vi "basic-main.vi"() -> ()   [LabVIEW 2015]
uses:
  states-enum.ctl
  Rack/Methods/Rack-Stop.vi
  Device/Methods/Lickometer-Stop.vi
  Rack/Typedefs/OutputRequest.ctl
  Rack/Typedefs/OutputRequest refnum.ctl
  Rack/Methods/Port drivers/DigitalInput-DataCluster.ctl
  Rack/Typedefs/InputData cluster.ctl
  Device/Typedefs/Lickometer.ctl
  Device/Typedefs/Speaker.ctl
  Device/Typedefs/Juicer.ctl
  Device/Typedefs/Valve.ctl
panel:
  in  "stop":bool
  out "Acc":dbl
  out "Time":dbl format="%#.0f"
  out "Trials":string
  out "Reward Dispensed (uL)":string
  out "Licks":string
  out "CR":string
  out "Miss":string
  out "FA":string
  out "Hits":string
  out "Current State":string
  out "Time Elapsed":dbl format="%<%H:%M:%S>t"
  in  "Tab Control":enum32{"Required", "Optional", "Devices"}(tab)
  in  "Tone Pairs":u16(ring) items=["1: CS+ 10000 Hz, CS- 5000 Hz", "2: CS+ 5800 Hz, CS- 5000 Hz", "3: CS+ 5000 Hz, CS- 10000 Hz", "4: CS+ 8000 Hz, CS- 15000 Hz"]
  in  "Max Time (s)":dbl=3600.0
  in  "Number of trials":string(combo)="200"
  in  "Max number of \nconsecutive trials":string(combo)="3"
  in  "Animal Name":string="Mouse"
  in  "Reward Vol. (uL)":dbl=5.0
  in  "Sequence Directory":path=path "C:/Users/SiapasLab/Desktop/git/wheatley"
  in  "Assay Description":string="Two Choice Audio Discrimination"
  in  "Recording Location":string="BI Room 146"
  in  "Trial delay (ms)":dbl=2000.0
  in  "Punish Time (s)":dbl=25.0
  in  "Trial window (ms)":dbl=3000.0
  in  "ITI lower (s)":dbl=8.0
  in  "ITI upper (s)":dbl=25.0
  in  "Min Licks":i32=1 min=1
  in  "Data Saving Directory":path=path "\\\\CA1-17\\ld8007/anesthesia/data"
  in  "Lickometer":T1={"Settings"={"Min lick duration"=1, "Port name"="bnc_panel.p0.3", "Port index"=0}, "Lick"=FALSE, "Debouncing"={"Semaphore"=refnum, "Lick start"=0}, "OutputRequest event ref"=refnum, "InputData reference"=refnum, "Active hi?"=FALSE}
  out "InputData":T4
  in  "Speaker":T6={"Settings"={"Portname"="BNC_Panel.ao0", "Index"=0, "Timestamp portname"="BNC_Panel.P0.0"}, "OutputRequest event ref"=refnum, "InputData reference"=refnum}
  in  "Juicer":T7={"Mode"=enum."Juice/reward", "Settings"={"Bleed #1 port index"=1, "Bleed #1 port name"="juicer.bleed1", "Bleed #2 port name"="juicer.bleed2", "Bleed #2 port index"=2, "Flush port name"="juicer.flush", "Flush port index"=3, "Purge port name"="juicer.purge", "Purge port index"=0, "Timestamp port name"="dsub_panel.p9.7"}, "OutputRequest event ref"=refnum, "InputData reference"=refnum}
  in  "Valve":T8={"Settings"={"Timestamp port name"="BNC_panel.P0.0", "Port name"="BNC_panel.P0.1", "Port index"=4}, "OutputRequest event ref"=refnum, "InputData reference"=refnum, "Default length (ms)"=100}
  # "(must be on same NI card)"
  # "(must be on same NI card)"
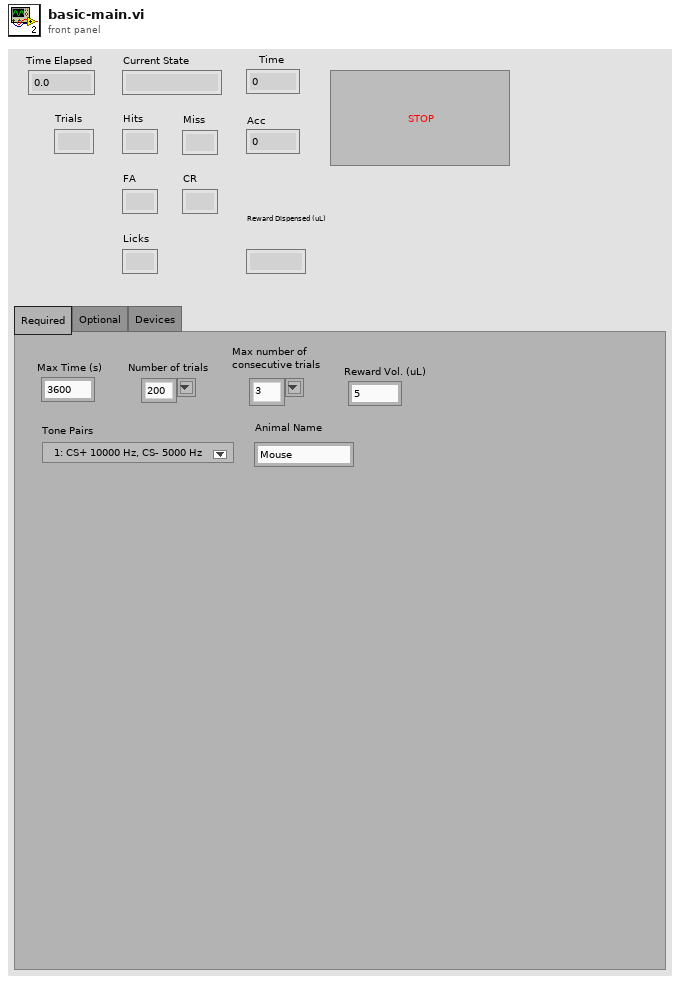
[diagram p1: front panel]
types:
  T1 = typedef "Lickometer.ctl" = cluster{"Settings":cluster{"Min lick duration":u32, "Port name":string, "Port index":i32}, "Lick":bool, "Debouncing":cluster{"Semaphore":T2, "Lick start":u32}, "OutputRequest event ref":T3, "InputData reference":refnum<vi>, "Active hi?":bool}
  T2 = typedef "Semaphore RefNum" = refnum<k1>
  T3 = typedef "OutputRequest refnum.ctl" = refnum<user-event>
  T4 = typedef "InputData cluster.ctl" = cluster{"DigitalInput":T5}
  T5 = typedef "DigitalInput-DataCluster.ctl" = cluster{"Falling":bool[], "Rising":bool[], "State":bool[]}
  T6 = typedef "Speaker.ctl" = cluster{"Settings":cluster{"Portname":string, "Index":i32, "Timestamp portname":string}, "OutputRequest event ref":T3, "InputData reference":refnum<vi>}
  T7 = typedef "Juicer.ctl" = cluster{"Mode":enum16{"Off", "Juice/reward", "Water flush", "Air purge"}, "Settings":cluster{"Bleed #1 port index":i32, "Bleed #1 port name":string, "Bleed #2 port name":string, "Bleed #2 port index":i32, "Flush port name":string, "Flush port index":i32, "Purge port name":string, "Purge port index":i32, "Timestamp port name":string}, "OutputRequest event ref":T3, "InputData reference":refnum<vi>}
  T8 = typedef "Valve.ctl" = cluster{"Settings":cluster{"Timestamp port name":string, "Port name":string, "Port index":i32}, "OutputRequest event ref":T3, "InputData reference":refnum<vi>, "Default length (ms)":i32}
  T9 = typedef "states-enum.ctl" = enum16{"ITI", "Trial", "Stop"}
  T10 = cluster{"ITI upper (s)":dbl, "ITI lower (s)":dbl, "Punish Time (s)":dbl, "Trial window (ms)":dbl, "Trial delay (ms)":dbl, "Max Time (s)":dbl, "Min Licks":i32, "Reward Vol. (uL)":dbl, "CS+ Tone":i32, "CS- Tone":i32}
  T11 = cluster{"appended path":path, "relative seconds":dbl, "Current Trial Index":i32, "Accuracy":dbl, "Hits":i32, "Miss":i32, "False Alarm":i32, "Correct Rejection":i32, "Licks":i32, "Reward Dispensed":dbl, "Punish ITI":bool, "Next Trial":i32}
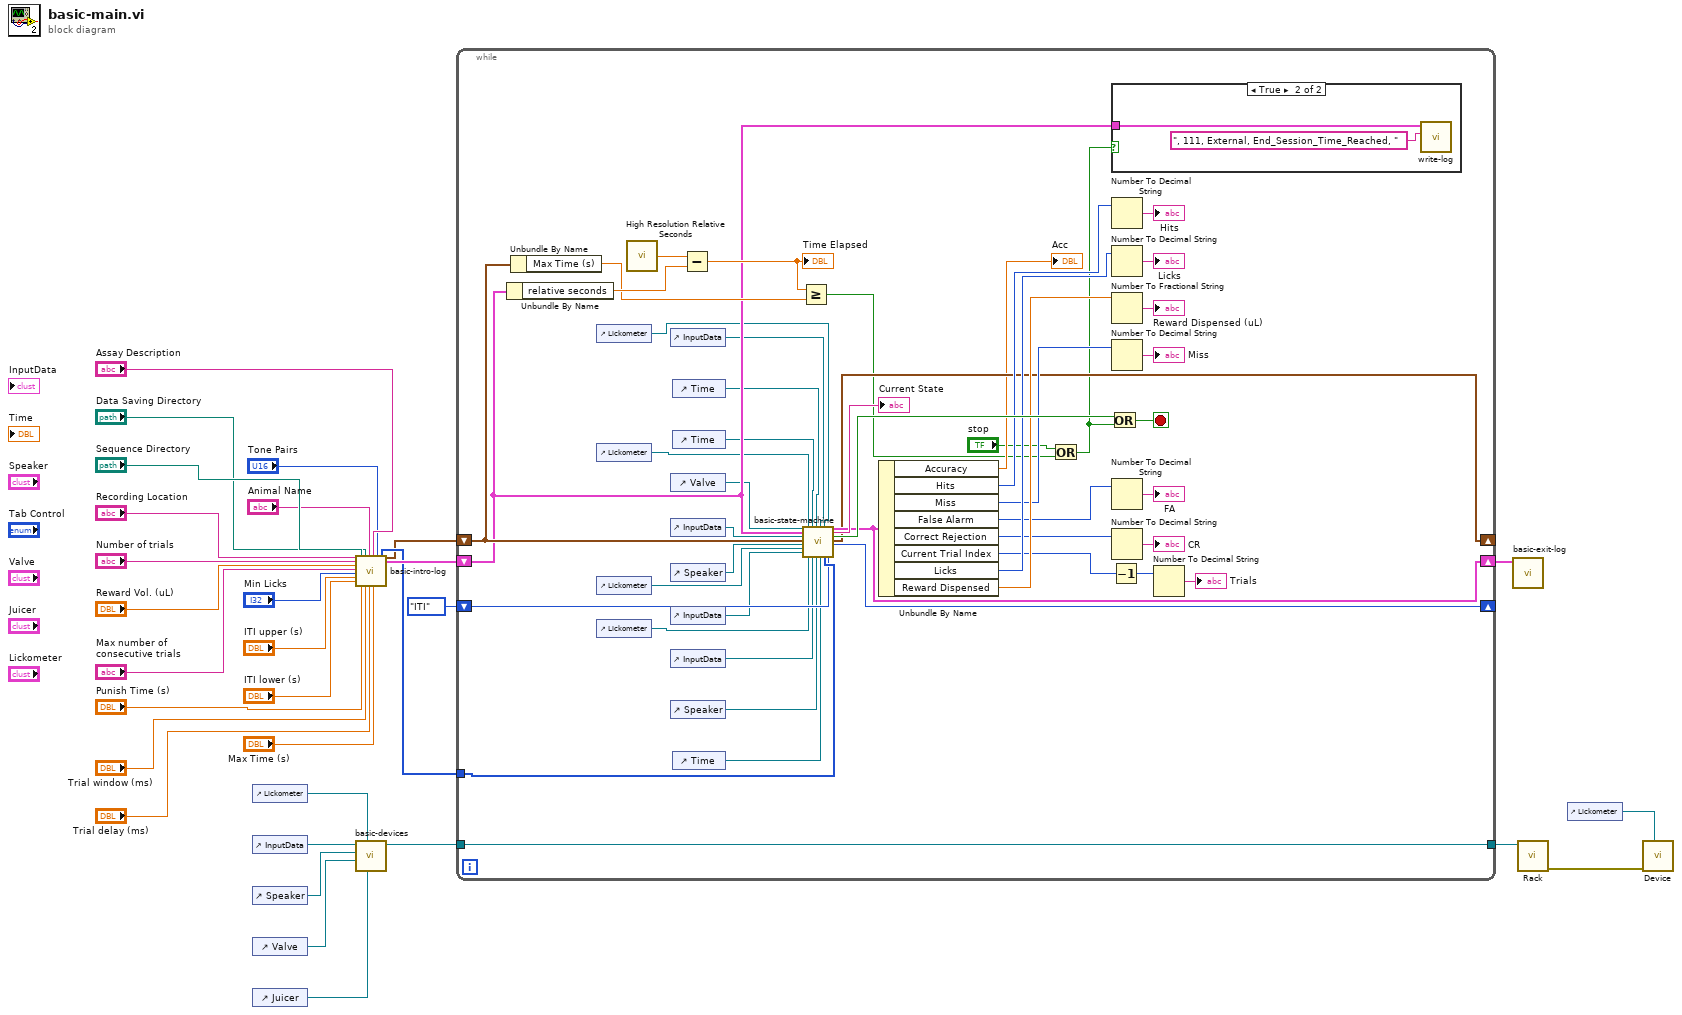
[diagram p0: block diagram]
diagram:
  n1 = control-ref of="Lickometer"() -> (w8:refnum<vi>)
  n2 = control-ref of="InputData"() -> (w3:refnum<vi>)
  n3 = control-ref of="Speaker"() -> (w4:refnum<vi>)
  n4 = control-ref of="Valve"() -> (w1:refnum<vi>)
  n5 = control-ref of="Juicer"() -> (w2:refnum<vi>)
  n6 = call "basic-intro-log.vi"("Recording Location"="Recording Location", "Number of trials"="Number of trials", "Reward Vol. (uL)"="Reward Vol. (uL)", "Max number of \nconsecutive trials"="Max number of \nconsecutive trials", "Min Licks"="Min Licks", "ITI upper (s)"="ITI upper (s)", "ITI lower (s)"="ITI lower (s)", "Sequence Directory"="Sequence Directory", "Punish Time (s)"="Punish Time (s)", "Data Saving Directory"="Data Saving Directory", "Trial window (ms)"="Trial window (ms)", "Animal Name"="Animal Name", "Trial delay (ms)"="Trial delay (ms)", "Assay Description"="Assay Description", "Max Time (s)"="Max Time (s)", "Tone Pairs"="Tone Pairs") -> ("all rows"=w16:i64[], "Cluster"=w14:T10, "Cluster 2"=w17:T11)  [unwired: 9 in]
  n7 = call "basic-devices.vi"("Juicer"=w2, "Lickometer"=w8, "Valve"=w1, "Speaker"=w4, "Cluster in"=w3) -> ("User Event out"=w6:T3)  [unwired: 6 in]
  n8 = while {
    shift-right: [w78] -> _
    shift-left: states-enum."ITI" -> [w55]
    shift-right: [w54] -> _
    shift-left: w14 -> [w70]
    shift-right: [w69] -> w13
    shift-left: w17 -> [w49]
    tunnel: w16 -> [w72]
    tunnel: w6 -> [w48]
    tunnel: [w48] -> w5
    stop <- w50 stop-if-true
    n9 = Unbundle By Name(w49) -> ("relative seconds"=w76:dbl)
    n10 = Unbundle By Name(w70) -> ("Max Time (s)"=w75:dbl)
    n11 = control-ref of="Lickometer"() -> (w43:refnum<vi>)
    n12 = control-ref of="Lickometer"() -> (w39:refnum<vi>)
    n13 = control-ref of="Lickometer"() -> (w36:refnum<vi>)
    n14 = control-ref of="Lickometer"() -> (w34:refnum<vi>)
    n15 = call <vilib>:"High Resolution Relative Seconds.vi"() -> ("relative seconds"=w77:dbl)
    n16 = control-ref of="InputData"() -> (w42:refnum<vi>)
    n17 = control-ref of="Valve"() -> (w44:refnum<vi>)
    n18 = control-ref of="InputData"() -> (w38:refnum<vi>)
    n19 = control-ref of="Speaker"() -> (w37:refnum<vi>)
    n20 = control-ref of="InputData"() -> (w35:refnum<vi>)
    n21 = control-ref of="InputData"() -> (w33:refnum<vi>)
    n22 = control-ref of="Speaker"() -> (w32:refnum<vi>)
    n23 = control-ref of="Time"() -> (w41:refnum<vi>)
    n24 = control-ref of="Time"() -> (w40:refnum<vi>)
    n25 = control-ref of="Time"() -> (w31:refnum<vi>)
    n26 = Subtract(x=w77, y=w76) -> (x-y=w73:dbl)
    "Time Elapsed" <- w73
    n27 = Greater Or Equal?(x=w73, y=w75) -> (x >= y?=w47:bool)
    n28 = call "basic-state-machine.vi"("Cluster in"=w44, "Cluster 2"=w49, "InputData 3"=w38, "Cluster 4"=w70, "Speaker"=w37, "Lickometer 2"=w36, "InputData 2"=w35, "Lickometer 3"=w39, "Lickometer"=w34, "Time 3"=w40, "InputData"=w33, "Time 2"=w41, "Speaker 2"=w32, "InputData 4"=w42, "Time"=w31, "Lickometer 4"=w43, "all rows"=w72, "Enum in"=w55) -> ("Cluster 3"=w69:T11, "String"=→"Current State":string, "Boolean"=w74:bool, "Cluster"=w54:T10, "Enum out"=w78:T9)  [unwired: 5 in]
    n29 = Unbundle By Name(w69) -> ("Accuracy"=→"Acc":dbl, "Hits"=w56:i32, "Miss"=w57:i32, "False Alarm"=w58:i32, "Correct Rejection"=w59:i32, "Current Trial Index"=w52:i32, "Licks"=w60:i32, "Reward Dispensed"=w61:dbl)
    n30 = Or(x="stop", y=w47) -> (x .or. y?=w45:bool)
    n31 = Or(x=w74, y=w45) -> (x .or. y?=w50:bool)
    n32 = Decrement(x=w52) -> (x-1=w53:i32)
    n33 = case shown="True" w45 {
      tunnel: w49 -> [_ w79]
      frame False {
      }
      frame True {
        n34 = call "write-log.vi"("Write Text"=", 111, External, End_Session_Time_Reached, " ("text"), "Internal Cluster"=w79) -> ()  [unwired: 10 in]
      }
    }
    n35 = Number To Decimal String(number=w56) -> (decimal integer string=→"Hits":string)  [unwired: 1 in]
    n36 = Number To Decimal String(number=w60) -> (decimal integer string=→"Licks":string)  [unwired: 1 in]
    n37 = Number To Fractional String(number=w61) -> (F-format string=→"Reward Dispensed (uL)":string)  [unwired: 3 in]
    n38 = Number To Decimal String(number=w57) -> (decimal integer string=→"Miss":string)  [unwired: 1 in]
    n39 = Number To Decimal String(number=w58) -> (decimal integer string=→"FA":string)  [unwired: 1 in]
    n40 = Number To Decimal String(number=w59) -> (decimal integer string=→"CR":string)  [unwired: 1 in]
    n41 = Number To Decimal String(number=w53) -> (decimal integer string=→"Trials":string)  [unwired: 1 in]
  }
  n42 = call "basic-exit-log.vi"("Cluster"=w13) -> ()  [unwired: 11 in]
  n43 = call-poly "Rack.vi"("OutputRequest channel"=w5) -> ("error out"=w9:errorcluster)  [unwired: 10 in]
  n44 = control-ref of="Lickometer"() -> (w7:refnum<vi>)
  n45 = call-poly "Device.vi"("Device reference"=w7, "error in (no error)"=w9) -> ()  [unwired: 9 in, 1 out]
